vi "sendCmdStatus.vi"(8 "error in (no error)":errorcluster, 9 "cmdStatus":string(combo)="ack", 10 "tcpPacket":T1, 11 "user event":refnum<user-event>) -> (0 "error out":errorcluster)   [LabVIEW 2018, in "TcpServerCmd.lvclass"]
doc: "Send Cmd Status to the TCP Server to inform the TCP Client about the command result."
uses:
  TcpServerCmd.lvclass
  typedef/ackTypeDef.ctl
  TcpServerBase/typedef/tcpPacketTypeDef.ctl
  TcpServerBase/TcpServerBase.lvclass
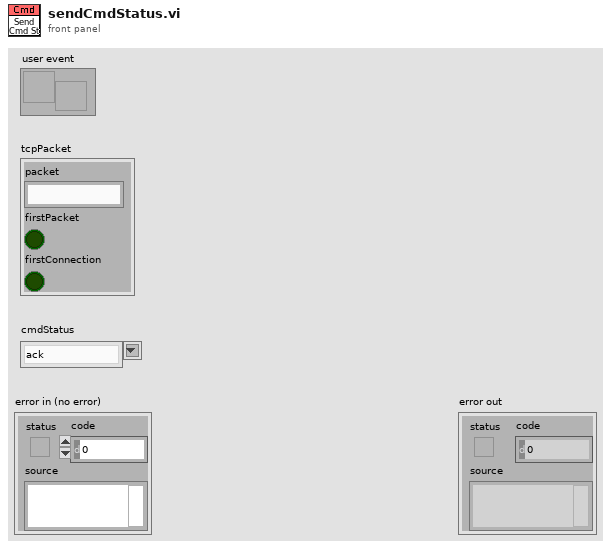
[diagram p1: front panel]
types:
  T1 = typedef "TcpServerBase.lvclass/tcpPacketTypeDef.ctl" = cluster{"packet":string, "firstPacket":bool, "firstConnection":bool}
  T2 = typedef "TcpServerCmd.lvclass/ackTypeDef.ctl" = cluster{"tcpPacket":T1, "cmdStatus":string}
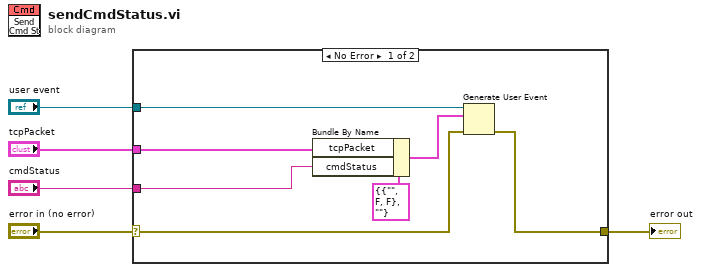
[diagram p0: block diagram]
diagram:
  n1 = case shown="No Error" "error in (no error)" {
    selector: "error in (no error)" -> [w8 w13]
    tunnel: [w10 w13] -> w4
    tunnel: "cmdStatus" -> [w11 _]
    tunnel: "user event" -> [w9 _]
    tunnel: "tcpPacket" -> [w7 _]
    frame No Error {
      n2 = Bundle By Name(cluster=T2 {"tcpPacket"={"packet"="", "firstPacket"=FALSE, "firstConnection"=FALSE}, "cmdStatus"=""} ("ack"), "tcpPacket"=w7, "cmdStatus"=w11) -> (w12:T2)
      n3 = Generate User Event(user event=w9, event data cluster=w12, error in=w8) -> (error out=w10:errorcluster)  [unwired: 1 in, 1 out]
    }
    frame Error {
    }
  }
  "error out" <- w4
